vi "Turret-firstVI.vi"(0 "MotorControlDevRef":T2={"DeviceStatus"={"status"=FALSE, "code"=0, "source"=""}, "Type"=enum."PWM", "PWM"={"PWM Channel"=enum."Invalid", "DeadBand"={"Name"="", "maxPositivePwm"=0, "minPositivePwm"=0, "centerPwm"=0, "maxNegativePwm"=0, "minNegativePwm"=0, "angularRange"=0}}, "CAN"={"Device Number"=0, "SetOutput VI Ref"=variant(enum8{"Percent VBus", "Current", "Speed", "Position", "Voltage"} enum."Percent VBus"), "GetOutput VI Ref"=variant(refnum<k1> refnum), "Enable VI Ref"=variant(dbl 12.0), "Disable VI Ref"=variant(enum8{"Percent VBus", "Speed", "Position", "Slave", "Unchanged / Invalid"} enum."Percent VBus"), "Data"=variant}, "Invert"=FALSE}, 1 "Current angle":dbl, 2 "desired Angle":dbl, 3 "PID Values":T1, 6 "Manual":bool, 7 "Feed CCW":dbl, 8 "Output":dbl, 9 "Feed CW":dbl, 10 "reinitialize? (F)":bool, 12 "Climbing?":bool) -> (14 "Motor Output":dbl)   [LabVIEW 2016]
uses:
  <vilib>/Rock Robotics/WPI/MotorControl/WPI_MotorControlDeviceRef.ctl
  <vilib>/Rock Robotics/WPI/MotorControl/WPI_MotorControlType.ctl
  <vilib>/Rock Robotics/SystemInterfaces/DIO/FPGA_DIOPWMChannel.ctl
  <vilib>/Rock Robotics/WPI/PWM/WPI_PWMDeadband.ctl
  <vilib>/addons/control/pid/pid.llb/PID (DBL).vi
  <vilib>/addons/control/pid/NI_PID_pid.lvlib
panel:
  in  "shooter range":dbl=90.0 format="%#_13g"
  in  "Softstop":dbl
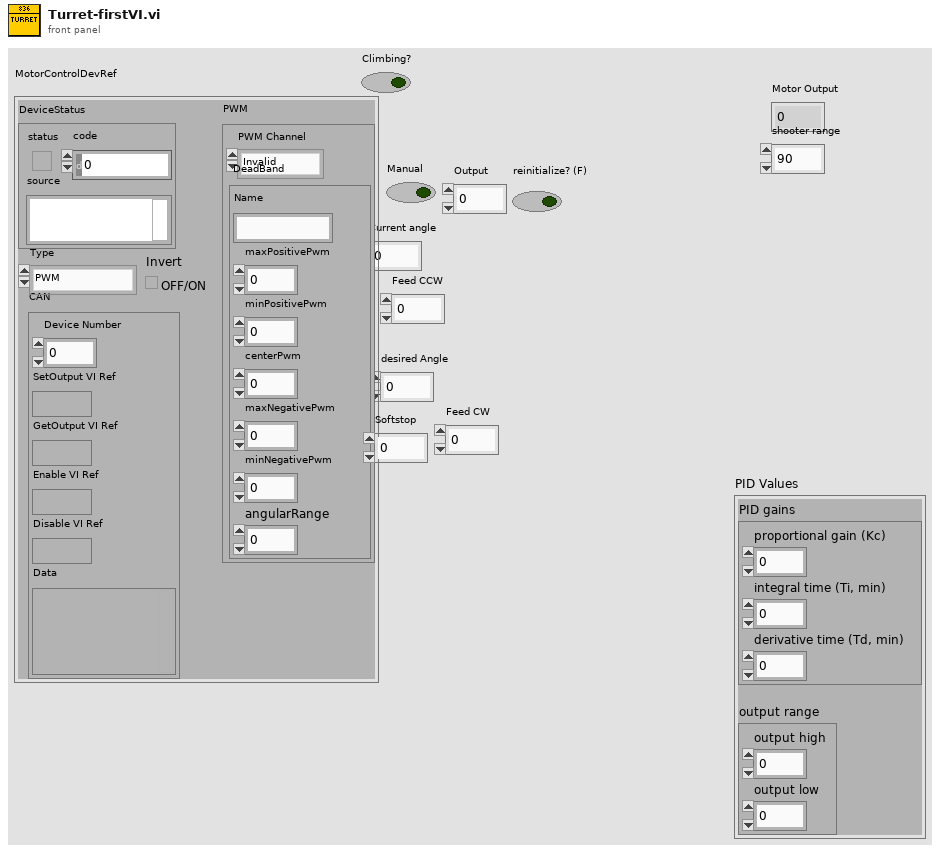
[diagram p1: front panel]
types:
  T1 = cluster{"PID gains":cluster{"proportional gain (Kc)":dbl, "integral time (Ti, min)":dbl, "derivative time (Td, min)":dbl}, "output range":cluster{"output high":dbl, "output low":dbl}}
  T2 = typedef "WPI_MotorControlDeviceRef.ctl" = cluster{"DeviceStatus":errorcluster, "Type":T3, "PWM":cluster{"PWM Channel":T4, "DeadBand":T5}, "CAN":cluster{"Device Number":u8, "SetOutput VI Ref":variant, "GetOutput VI Ref":variant, "Enable VI Ref":variant, "Disable VI Ref":variant, "Data":variant}, "Invert":bool}
  T3 = typedef "WPI_MotorControlType.ctl" = enum16{"PWM", "CAN"}
  T4 = typedef "FPGA_DIOPWMChannel.ctl" = enum8{"PWM 0", "PWM 1", "PWM 2", "PWM 3", "PWM 4", "PWM 5", "PWM 6", "PWM 7", "PWM 8", "PWM 9", "PWM MXP 0", "PWM MXP 1", "PWM MXP 2", "PWM MXP 3", "PWM MXP 4", "PWM MXP 5", "PWM MXP 6", "PWM MXP 7", "PWM MXP 8", "PWM MXP 9", "Invalid"}
  T5 = typedef "WPI_PWMDeadband.ctl" = cluster{"Name":string, "maxPositivePwm":i32, "minPositivePwm":i32, "centerPwm":i32, "maxNegativePwm":i32, "minNegativePwm":i32, "angularRange":u16}
  T6 = cluster{"proportional gain (Kc)":dbl, "integral time (Ti, min)":dbl, "derivative time (Td, min)":dbl}
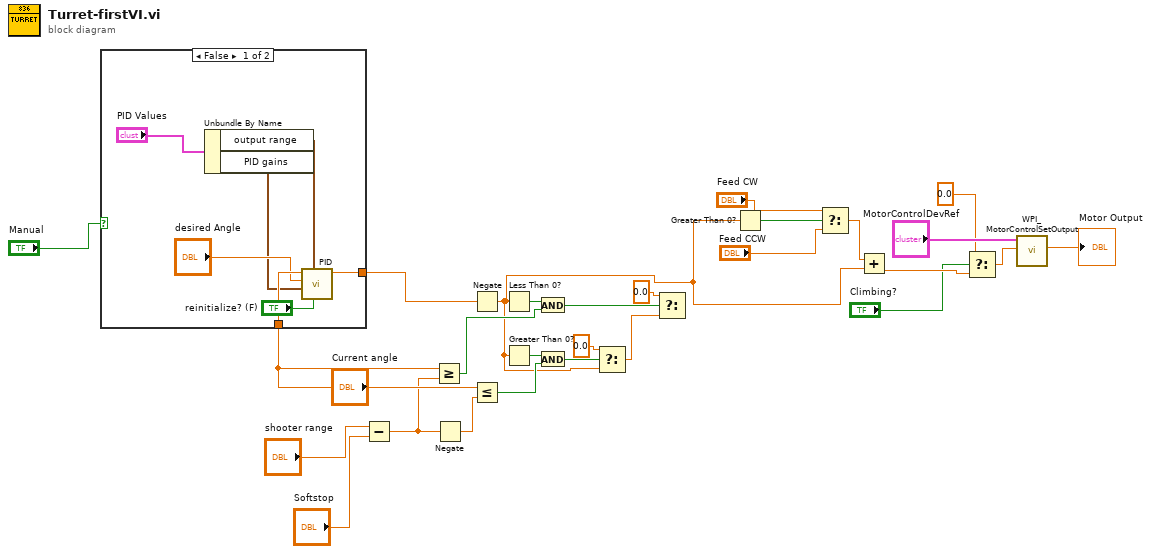
[diagram p0: block diagram]
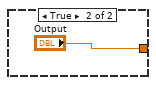
[diagram p2: hidden frame]
diagram:
  n1 = case shown="False" "Manual" {
    tunnel: "Current angle" -> [w34 _]
    tunnel: [w32 "Output"] -> w12
    frame False {
      n2 = Unbundle By Name("PID Values") -> ("output range"=w29:cluster{"output high":dbl, "output low":dbl}, "PID gains"=w28:T6)
      n3 = call-poly <vilib>:"PID.vi"("reinitialize? (F)"="reinitialize? (F)", "output range"=w29, "PID gains"=w28, "process variable"="desired Angle", "setpoint"=w34) -> ("output"=w32:dbl)  [unwired: 5 in, 1 out]
    }
    frame True {
    }
  }
  n4 = Subtract(x="shooter range", y="Softstop") -> (x-y=w14:dbl)
  n5 = Greater Or Equal?(x="Current angle", y=w14) -> (x >= y?=w24:bool)
  n6 = Negate(x=w14) -> (-x=w23:dbl)
  n7 = Negate(x=w12) -> (-x=w5:dbl)
  n8 = Less Or Equal?(x="Current angle", y=w23) -> (x <= y?=w20:bool)
  n9 = Less Than 0?(x=w5) -> (x < 0?=w16:bool)
  n10 = Greater Than 0?(x=w5) -> (x > 0?=w17:bool)
  n11 = And(x=w16, y=w24) -> (x .and. y?=w21:bool)
  n12 = And(x=w17, y=w20) -> (x .and. y?=w22:bool)
  n13 = Select(t=0.0, s=w22, f=w5) -> (s? t:f=w25:dbl)
  n14 = Select(t=0.0, s=w21, f=w25) -> ()  [unwired: 1 out]
  n15 = Greater Than 0?(x=w5) -> (x > 0?=w6:bool)
  n16 = Select(t="Feed CW", s=w6, f="Feed CCW") -> (s? t:f=w7:dbl)
  n17 = Add(x=w7, y=w5) -> (x+y=w3:dbl)
  n18 = Select(t=0.0, s="Climbing?", f=w3) -> (s? t:f=w4:dbl)
  n19 = call <vilib>:"WPI_MotorControlSetOutput.vi"("Output"=w4, "MotorControlDevRef"="MotorControlDevRef") -> ("Motor Output"=→"Motor Output":dbl)  [unwired: 7 in, 2 out]
